vi "SQL Fetch Data (GetString).vi"(8 "error in (no error)":errorcluster, 11 "ADODB._Recordset In":refnum<k7>) -> (0 "error out":errorcluster, 1 "ADODB._Recordset Out":refnum<k7>, 2 "Rows Fetched":i32, 3 "Data":string[][](array[string]))   [LabVIEW 2011]
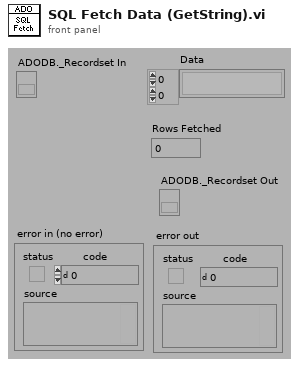
[diagram p1: front panel]
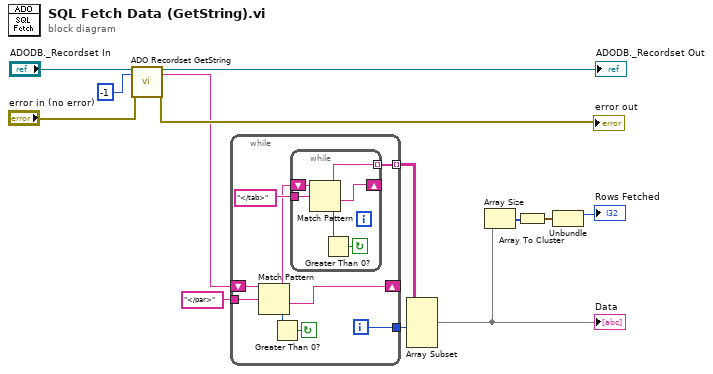
[diagram p0: block diagram]
diagram:
  n1 = call <userlib>:"ADO Recordset GetString.vi"("ADODB._Recordset"="ADODB._Recordset In", "NumRows"=-1, "error in (no error)"="error in (no error)") -> ("ADODB._Recordset Out"=→"ADODB._Recordset Out":refnum<k7>, "GetString"=w2:string, "error out"=→"error out":errorcluster)  [unwired: 14 in]
  n2 = while {
    tunnel: [w17] -> w3 mode=indexing
    tunnel: [w20] -> w5
    tunnel: "</par>" ("delimiter (Tab)") -> [w22]
    shift-right: [w15] -> _
    shift-left: w2 -> [w16]
    i -> [w20]
    stop <- w21 continue-if-true
    n3 = Match Pattern(string=w16, regular expression=w22) -> (before substring=w14:string, after substring=w15:string, offset past match=w19:i32)  [unwired: 1 in, 1 out]
    n4 = Greater Than 0?(x=w19) -> (x > 0?=w21:bool)
    n5 = while {
      shift-right: [w27] -> _
      shift-left: w14 -> [w28]
      tunnel: [w26] -> w17 mode=indexing
      tunnel: "</tab>" ("delimiter (Tab)") -> [w23]
      stop <- w25 continue-if-true
      n6 = Match Pattern(string=w28, regular expression=w23) -> (before substring=w26:string, after substring=w27:string, offset past match=w24:i32)  [unwired: 1 in, 1 out]
      n7 = Greater Than 0?(x=w24) -> (x > 0?=w25:bool)
    }
  }
  n8 = Array Subset(array=w3, length (row)=w5) -> (w1:string[][])  [unwired: 3 in]
  "Data" <- w1
  n9 = Array Size(array=w1) -> (size(s)=w13:i32[])
  n10 = Array To Cluster(array=w13) -> (cluster=w12:cluster{"[0]":i32, "[1]":i32})
  n11 = Unbundle(w12) -> ("[0]"=→"Rows Fetched":i32)  [unwired: 1 out]
